vi "Send RegisterByLabel.vi"(8 "error in (no error)":errorcluster, 9 "Observer to Register":refnum<class "Send.lvclass">, 10 "Label":string, 11 "MSR Parent in":refnum<class "Send.lvclass">) -> (0 "error out":errorcluster, 3 "MSR Parent out":refnum<class "Send.lvclass">)   [LabVIEW 2011, in "Messenging.lvlib" / "ObserverRegistry.lvclass"]
uses:
  ObserverRegistry.lvclass
  Interprocess Messenger/Send/Send.lvclass
  Commands/Register by Label/Observer_RegisterByLabel.lvclass
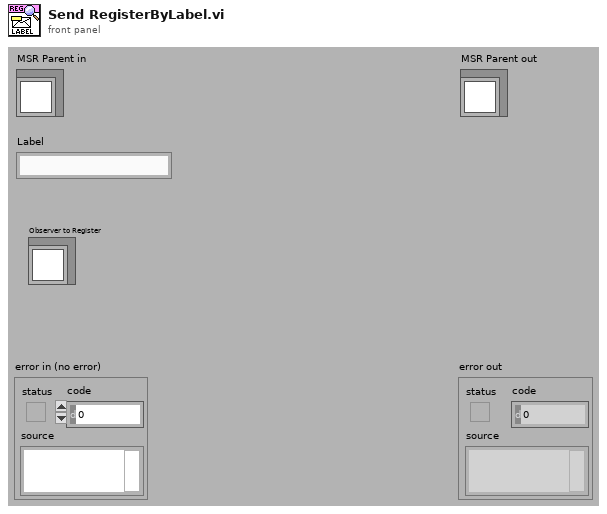
[diagram p1: front panel]
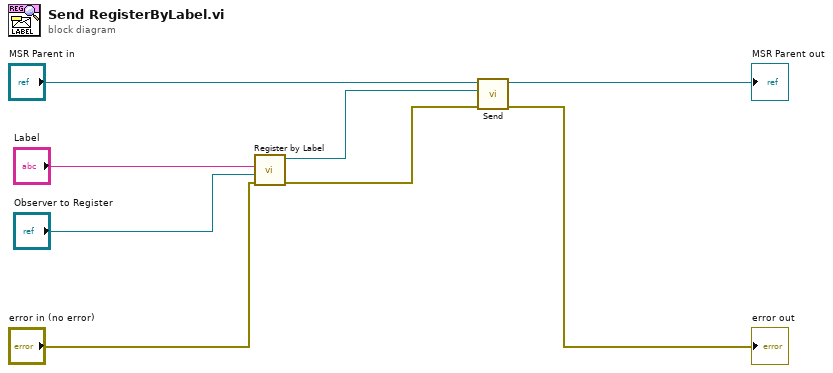
[diagram p0: block diagram]
diagram:
  n1 = call "Register by Label.vi"("error in (no error)"="error in (no error)", "Observer"="Observer to Register", "Label to Register For"="Label") -> ("error out"=w2:errorcluster, "ObserverRegistryCommand_RegisterByLabel out"=w1:refnum<class "Observer_RegisterByLabel.lvclass">)  [unwired: 7 out]
  n2 = call-dynamic "Send.vi"("error in (no error)"=w2, "Message"=w1, "MSR Parent in"="MSR Parent in") -> ("error out"=→"error out":errorcluster, "MSR Parent out"=→"MSR Parent out":refnum<class "Send.lvclass">)  [unwired: 7 out]
